vi "Text To Speech.vi"(8 "error in (no error)":errorcluster, 11 "textToSpeak":string="Hello and welcome to the Cambridge LabVIEW Users Group") -> (0 "error out":errorcluster)   [LabVIEW 2018]
doc: "<b>Speak Text.vi </b> - simple example of how to call the .NET speech synthesiser to speak a string of text.\n\nThoric\n2009\n\nNote: You can install additional voices to the speech synthesiser. These can be selected in the more advanced vi's.\nNote: The default voice of Mary under Windows VISTA/Win7 is more realistic than any of the voices available under Windows XP."
uses:
  System.Speech
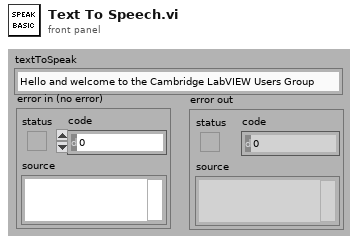
[diagram p1: front panel]
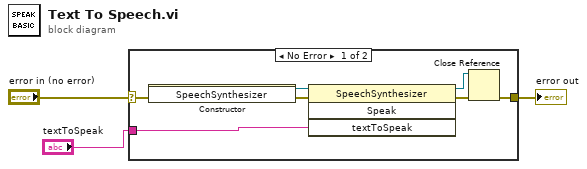
[diagram p0: block diagram]
diagram:
  n1 = case shown="No Error" "error in (no error)" {
    selector: "error in (no error)" -> [w5 w11]
    tunnel: "textToSpeak" -> [w6 _]
    tunnel: [w4 w11] -> w1
    frame No Error {
      n2 = constructor class="SpeechSynthesizer"(error in=w5) -> (reference out=w10:refnum<k24>, error out=w9:errorcluster)  [unwired: 2 in, 1 out]
      n3 = invoke class="SpeechSynthesizer" method="Speak"(reference=w10, error in=w9, "textToSpeak"=w6) -> (reference out=w7:refnum<k24>, error out=w8:errorcluster)  [unwired: 1 in, 2 out]
      n4 = Close Reference(reference=w7, error in (no error)=w8) -> (error out=w4:errorcluster)
    }
    frame Error {
    }
  }
  "error out" <- w1
